vi "CRYDV MARK.vi"(0 "sAction":string="asada", 1 "mVritual_VIRef":refnum<vi>, 2 "sData":string="asada", 3 "MousePos":T1, 4 "DataView Array Index":i32, 5 "SubPanel array":refnum<vi>[](array[refnum]), 6 "Start Pos In":T1) -> (10 "bResult":bool=TRUE)   [LabVIEW 2013]
uses:
  <vilib>/Utility/miscctls.llb/LVRectTypeDef.ctl
  CRYNew View Global.vi
panel:
  in  "Rect_Main":T2
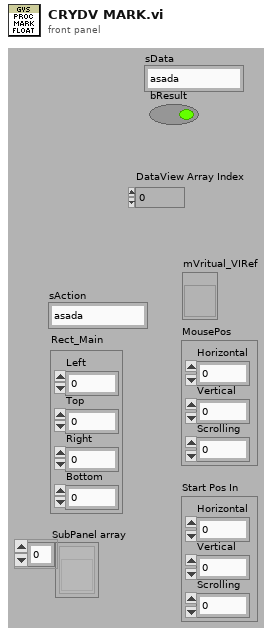
[diagram p1: front panel]
types:
  T1 = cluster{"Horizontal":i32, "Vertical":i32, "Scrolling":i32}
  T2 = typedef "LVRectTypeDef.ctl" = cluster{"Left":i16, "Top":i16, "Right":i16, "Bottom":i16}
  T3 = typedef "Graph Main Info Cluster.ctl" = cluster{"Selected_BarIdx":i32, "Selected_PanelIdx":i32, "Graph Main VIRef":refnum<vi>, "ToolBarClick":bool, "Spliter Ref Array":refnum<vi>[], "Panel Ref Array":refnum<vi>[], "Spliter_matrix":i32[][], "Panel_matrix":i32[][], "child_spliterIdx_matrix":i32[][], "split_pos_matrix":i32[][], "Title State":bool, "sQueueName":string, "Frame nID":i32, "Graph VIRef Array":cluster{"Graph VIRef":refnum<vi>, "Panel Idx":i32, "Frame VIRef":refnum<vi>, "Icon Ring":i32, "Graph Type":string}[], "View Type":string}
  T4 = enum32{"Invalid", "Standard", "Closed", "Hidden", "Minimized", "Maximized"}
  T5 = enum32{"Invalid", "Default", "Floating", "Floating/Auto-Hide", "Modal"}
  T6 = cluster{"Horizontal":bool, "Vertical":bool, "Scrolling":bool}
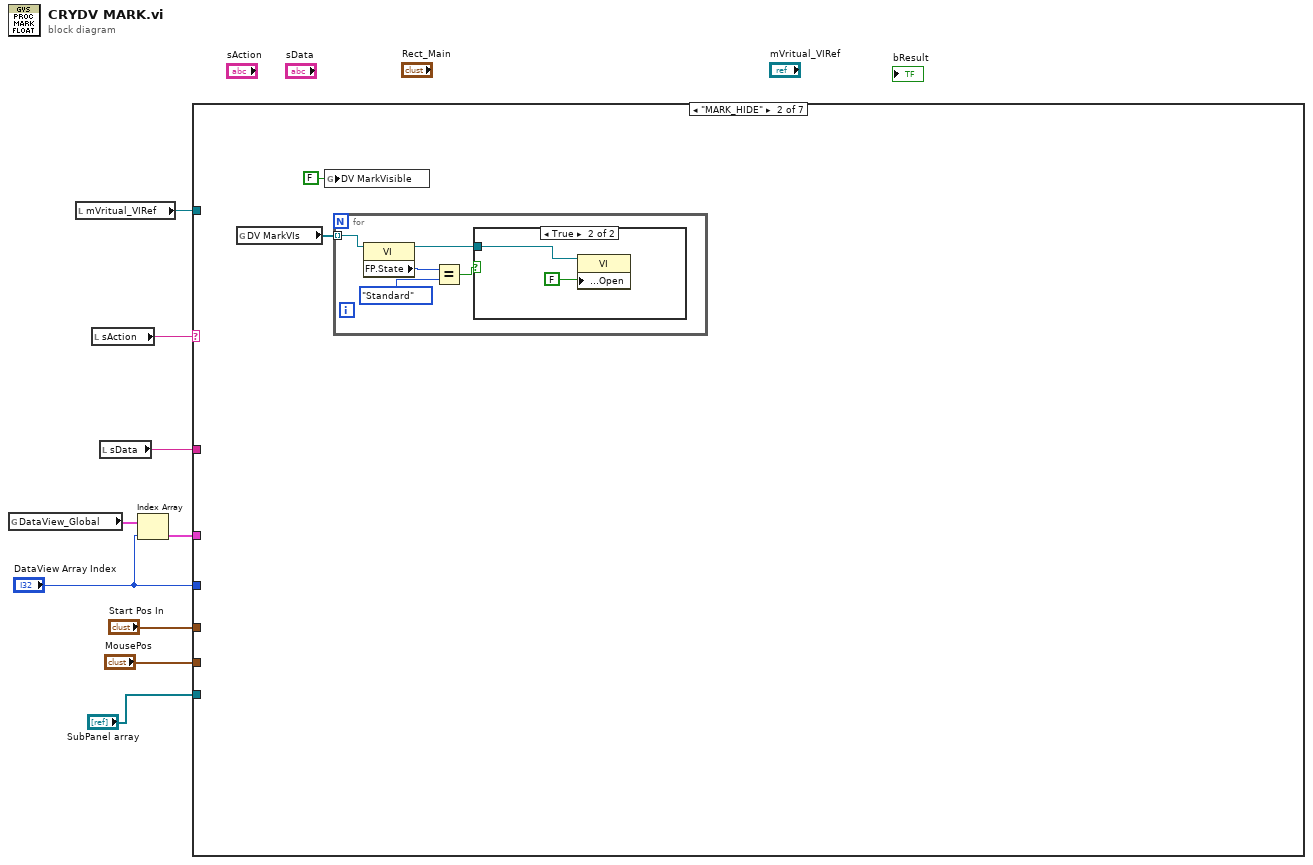
[diagram p0: block diagram]
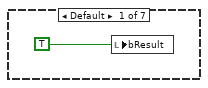
[diagram p2: hidden frame]
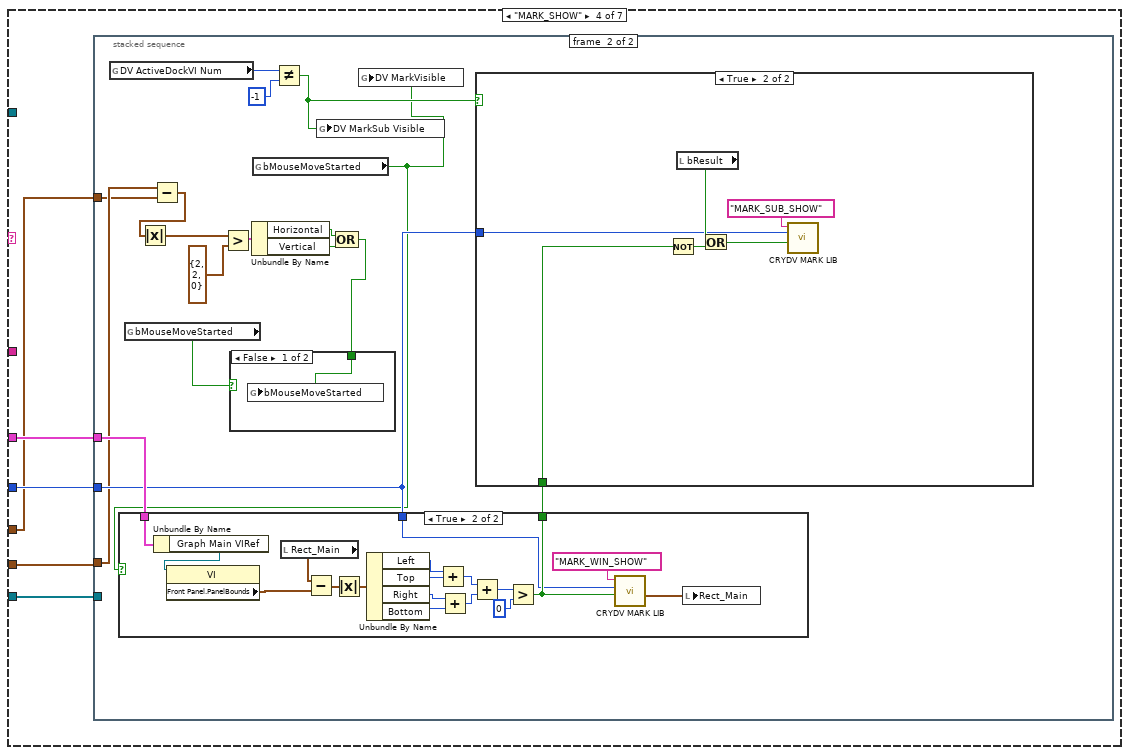
[diagram p5: hidden frame]
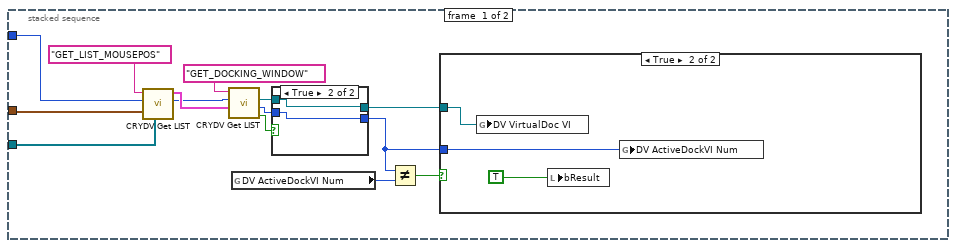
[diagram p6: hidden frame]
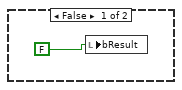
[diagram p7: hidden frame]
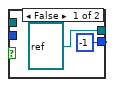
[diagram p8: hidden frame]
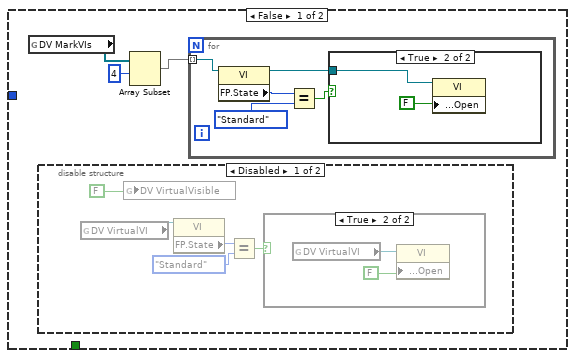
[diagram p11: hidden frame]
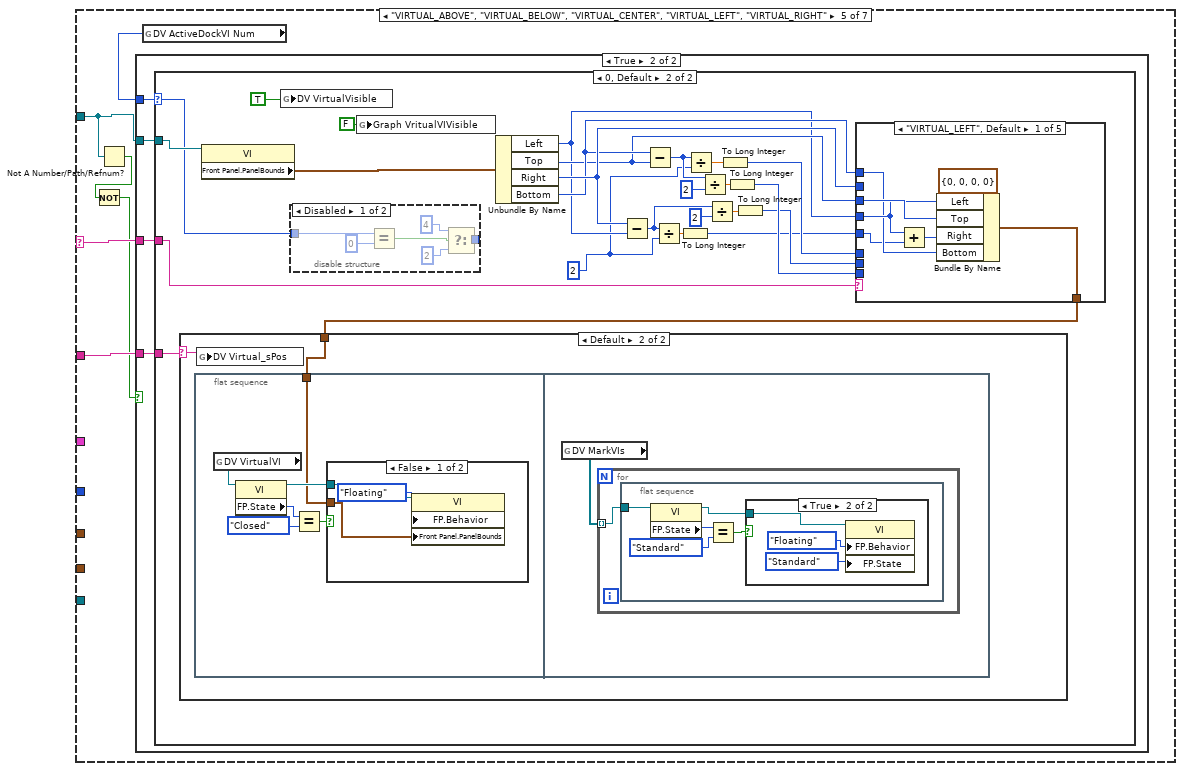
[diagram p15: hidden frame]
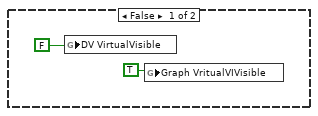
[diagram p16: hidden frame]
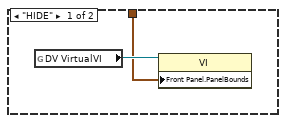
[diagram p19: hidden frame]
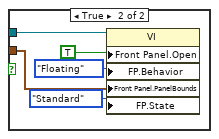
[diagram p20: hidden frame]
diagram:
  n1 = global read "CRYNew View Global.vi" "DataView_Global"() -> (w5:T3[])
  n2 = local read "mVritual_VIRef"() -> (w3:refnum<vi>)
  n3 = local read "sAction"() -> (w9:string)
  n4 = local read "sData"() -> (w8:string)
  n5 = Index Array(array=w5, index="DataView Array Index") -> (element=w7:T3)
  n6 = case shown="\"MARK_HIDE\"" w9 {
    selector: w9 -> [_ _ _ _ w110 _ _]
    tunnel: "MousePos" -> [_ _ _ w24 _ _ w223]
    tunnel: w3 -> [_ _ _ _ w107 _ _]
    tunnel: w8 -> [_ _ _ _ w109 _ _]
    tunnel: w7 -> [_ _ _ w23 _ _ _]
    tunnel: "DataView Array Index" -> [_ _ _ w22 _ _ _]
    tunnel: "SubPanel array" -> [_ _ _ w21 _ _ _]
    tunnel: "Start Pos In" -> [_ _ _ w20 _ _ _]
    frame Default {
      n7 = local write "bResult"(TRUE ("bResult")) -> ()
    }
    frame "MARK_HIDE" {
      n8 = global read "CRYNew View Global.vi" "DV MarkVIs"() -> (w12:refnum<vi>[])
      n9 = global write "CRYNew View Global.vi" "DV MarkVisible"(FALSE ("Mark VI State")) -> ()
      n10 = for {
        tunnel: w12 -> [w15] mode=indexing
        n11 = property class="VI"(reference=w15) -> (reference out=w14:refnum<vi>, "FP.State"=w17:T4)  [unwired: 1 in, 1 out]
        n12 = Equal?(x=w17, y=T4."Standard" ("Front Panel Window:State")) -> (x = y?=w13:bool)
        n13 = case shown="True" w13 {
          tunnel: w14 -> [_ w19]
          frame False {
          }
          frame True {
            n14 = property class="VI"(reference=w19, "Front Panel.Open"=FALSE ("Front Panel Window:Open")) -> ()  [unwired: 1 in, 2 out]
          }
        }
      }
    }
    frame "ADDGRAPHMENU_HIDE" {
    }
    frame "MARK_SHOW" {
      n15 = stacked-sequence {
        tunnel: w24 -> [w37 w50]
        tunnel: w23 -> [_ w59]
        tunnel: w22 -> [w26 w58]
        tunnel: w21 -> [w25 _]
        tunnel: w20 -> [_ w49]
        frame #0 {
          n16 = call "CRYDV Get LIST.vi"("sAction"="GET_LIST_MOUSEPOS", "DataView Array Index"=w26, "MousePos"=w37, "SubPanel array"=w25) -> ("List_Out"=w34:cluster{"nID":i32, "pVIRef":refnum<vi>}[])  [unwired: 1 in, 5 out]
          n17 = call "CRYDV Get LIST.vi"("sAction"="GET_DOCKING_WINDOW", "DataView Array Index"=w26, "List_In"=w34) -> ("pVIRef_Out"=w32:refnum<vi>, "nData_Out"=w29:i32, "bResult"=w33:bool)  [unwired: 2 in, 3 out]
          n18 = global read "CRYNew View Global.vi" "DV ActiveDockVI Num"() -> (w27:i32)
          n19 = case shown="True" w33 {
            tunnel: w32 -> [_ w45]
            tunnel: [-1 w44] -> w30
            tunnel: [refnum<vi> refnum ("Vritual_Docking_VIRef") w45] -> w31
            tunnel: w29 -> [_ w44]
            frame False {
            }
            frame True {
            }
          }
          n20 = Not Equal?(x=w30, y=w27) -> (x != y?=w28:bool)
          n21 = case shown="True" w28 {
            tunnel: w31 -> [_ w41]
            tunnel: w30 -> [_ w39]
            frame False {
              n22 = local write "bResult"(FALSE ("Docking_Update")) -> ()
            }
            frame True {
              n23 = global write "CRYNew View Global.vi" "DV VirtualDoc VI"(w41) -> ()
              n24 = local write "bResult"(TRUE ("Docking_Update")) -> ()
              n25 = global write "CRYNew View Global.vi" "DV ActiveDockVI Num"(w39) -> ()
            }
          }
        }
        frame #1 {
          n26 = global read "CRYNew View Global.vi" "DV ActiveDockVI Num"() -> (w61:i32)
          n27 = global read "CRYNew View Global.vi" "bMouseMoveStarted"() -> (w47:bool)
          n28 = Subtract(x=w50, y=w49) -> (x-y=w52:T1)
          n29 = Absolute Value(x=w52) -> (abs(x)=w51:T1)
          n30 = Greater?(x=w51, y=T1 {"Horizontal"=2, "Vertical"=2, "Scrolling"=0}) -> (0:w55:T6)
          n31 = Unbundle By Name(w55) -> ("Horizontal"=w54:bool, "Vertical"=w53:bool)
          n32 = global read "CRYNew View Global.vi" "bMouseMoveStarted"() -> (w48:bool)
          n33 = case shown="True" w48 {
            tunnel: [_ w66] -> w60
            tunnel: w59 -> [_ w65]
            tunnel: w58 -> [_ w64]
            frame False {
            }
            frame True {
              n34 = Unbundle By Name(w65) -> ("Graph Main VIRef"=w68:refnum<vi>)
              n35 = property class="VI"(reference=w68) -> ("Front Panel.PanelBounds"=w67:T2)  [unwired: 1 in, 2 out]
              n36 = local read "Rect_Main"() -> (w69:T2)
              n37 = Subtract(x=w69, y=w67) -> (x-y=w73:T2)
              n38 = Absolute Value(x=w73) -> (abs(x)=w72:T2)
              n39 = Unbundle By Name(w72) -> ("Left"=w74:i16, "Top"=w77:i16, "Right"=w76:i16, "Bottom"=w75:i16)
              n40 = Add(x=w74, y=w77) -> (x+y=w78:i16)
              n41 = Add(x=w76, y=w75) -> (x+y=w79:i16)
              n42 = Add(x=w78, y=w79) -> (x+y=w71:i16)
              n43 = Greater?(x=w71, y=0) -> (0:w66:bool)
              n44 = call "CRYDV MARK LIB.vi"("sAction"="MARK_WIN_SHOW", "DataView Array Index"=w64, "Docking_Update"=w66) -> ("Rect_Out"=w80:T2)  [unwired: 1 in, 6 out]
              n45 = local write "Rect_Main"(w80) -> ()
            }
          }
          n46 = Not Equal?(x=w61, y=-1) -> (x != y?=w57:bool)
          n47 = global write "CRYNew View Global.vi" "DV MarkSub Visible"(w57) -> ()
          n48 = Compound Arithmetic op=OR(w54, w53) -> (w46:bool)
          n49 = case shown="False" w47 {
            tunnel: w46 -> [w63 _]
            frame False {
              n50 = global write "CRYNew View Global.vi" "bMouseMoveStarted"(w63) -> ()
            }
            frame True {
            }
          }
          n51 = global write "CRYNew View Global.vi" "DV MarkVisible"(w48) -> ()
          n52 = case shown="True" w57 {
            tunnel: w60 -> [_ w100]
            tunnel: w58 -> [_ w99]
            frame False {
              n53 = global read "CRYNew View Global.vi" "DV MarkVIs"() -> (w84:refnum<vi>[])
              n54 = disable-structure shown="Disabled" {
                frame Disabled {
                  n55 = global read "CRYNew View Global.vi" "DV VirtualVI"() -> (w87:refnum<vi>)
                  n56 = global write "CRYNew View Global.vi" "DV VirtualVisible"(FALSE ("VirtualVi")) -> ()
                  n57 = property class="VI"(reference=w87) -> ("FP.State"=w88:T4)  [unwired: 1 in, 2 out]
                  n58 = Equal?(x=w88, y=T4."Standard" ("Front Panel Window:State")) -> (x = y?=w85:bool)
                  n59 = case shown="True" w85 {
                    frame False {
                    }
                    frame True {
                      n60 = global read "CRYNew View Global.vi" "DV VirtualVI"() -> (w90:refnum<vi>)
                      n61 = property class="VI"(reference=w90, "Front Panel.Open"=FALSE ("Front Panel Window:Open")) -> ()  [unwired: 1 in, 2 out]
                    }
                  }
                }
                frame Enabled {
                }
              }
              n62 = Array Subset(array=w84, index=4) -> (w83:refnum<vi>[])  [unwired: 1 in]
              n63 = for {
                tunnel: w83 -> [w94] mode=indexing
                n64 = property class="VI"(reference=w94) -> (reference out=w93:refnum<vi>, "FP.State"=w96:T4)  [unwired: 1 in, 1 out]
                n65 = Equal?(x=w96, y=T4."Standard" ("Front Panel Window:State")) -> (x = y?=w92:bool)
                n66 = case shown="True" w92 {
                  tunnel: w93 -> [_ w98]
                  frame False {
                  }
                  frame True {
                    n67 = property class="VI"(reference=w98, "Front Panel.Open"=FALSE ("Front Panel Window:Open")) -> ()  [unwired: 1 in, 2 out]
                  }
                }
              }
            }
            frame True {
              n68 = Not(x=w100) -> (.not. x?=w102:bool)
              n69 = local read "bResult"() -> (w103:bool)
              n70 = Or(x=w103, y=w102) -> (x .or. y?=w104:bool)
              n71 = call "CRYDV MARK LIB.vi"("sAction"="MARK_SUB_SHOW", "DataView Array Index"=w99, "Docking_Update"=w104) -> ()  [unwired: 1 in, 7 out]
            }
          }
        }
      }
    }
    frame "VIRTUAL_ABOVE", "VIRTUAL_BELOW", "VIRTUAL_CENTER", "VIRTUAL_LEFT", "VIRTUAL_RIGHT" {
      n72 = Not A Number/Path/Refnum?(number/path/refnum=w107) -> (NaN/Path/Refnum?=w106:bool)
      n73 = Not(x=w106) -> (.not. x?=w105:bool)
      n74 = global read "CRYNew View Global.vi" "DV ActiveDockVI Num"() -> (w108:i32)
      n75 = case shown="True" w105 {
        tunnel: w107 -> [_ w116]
        tunnel: w110 -> [_ w115]
        tunnel: w109 -> [_ w114]
        tunnel: w108 -> [_ w113]
        frame False {
          n76 = global write "CRYNew View Global.vi" "DV VirtualVisible"(FALSE ("Virtual_State_Up")) -> ()
          n77 = global write "CRYNew View Global.vi" "Graph VritualVIVisible"(TRUE ("VritualVIVisible")) -> ()
        }
        frame True {
          n78 = case shown="0, Default" w113 {
            selector: w113 -> [_ w120]
            tunnel: w115 -> [_ w130]
            tunnel: w116 -> [_ w140]
            tunnel: w114 -> [_ w121]
            frame -1 {
            }
            frame 0, Default {
              w118 = 2
              n79 = property class="VI"(reference=w140) -> ("Front Panel.PanelBounds"=w119:T2)  [unwired: 1 in, 2 out]
              n80 = global write "CRYNew View Global.vi" "DV VirtualVisible"(TRUE ("Virtual_State_Up")) -> ()
              n81 = disable-structure shown="Disabled" {
                disable-tunnel: [w145 _] -> _
                disable-tunnel: w120 -> [w142 _]
                frame Disabled {
                  n82 = Equal?(x=w142, y=0) -> (x = y?=w143:bool)
                  n83 = Select(t=4, s=w143, f=2) -> (s? t:f=w145:i32)
                }
                frame Enabled {
                }
              }
              n84 = global write "CRYNew View Global.vi" "Graph VritualVIVisible"(FALSE ("VritualVIVisible")) -> ()
              n85 = Unbundle By Name(w119) -> ("Left"=w132:i16, "Top"=w133:i16, "Right"=w139:i16, "Bottom"=w138:i16)
              n86 = Subtract(x=w139, y=w132) -> (x-y=w134:i16)
              n87 = Subtract(x=w138, y=w133) -> (x-y=w137:i16)
              n88 = Divide(x=w134, y=w118) -> (x/y=w123:dbl)
              n89 = To Long Integer(number=w123) -> (32bit integer=w122:i32)
              n90 = Divide(x=w137, y=w118) -> (x/y=w129:dbl)
              n91 = Divide(x=w137, y=2) -> (x/y=w127:dbl)
              n92 = Divide(x=w134, y=2) -> (x/y=w125:dbl)
              n93 = To Long Integer(number=w129) -> (32bit integer=w128:i32)
              n94 = To Long Integer(number=w127) -> (32bit integer=w126:i32)
              n95 = To Long Integer(number=w125) -> (32bit integer=w124:i32)
              n96 = case shown="\"VIRTUAL_LEFT\", Default" w130 {
                tunnel: w132 -> [w180 _ w194 w201 w216]
                tunnel: w133 -> [w181 w188 w193 _ w215]
                tunnel: w139 -> [_ w186 w195 w202 _]
                tunnel: w138 -> [w178 w187 _ w199 _]
                tunnel: w122 -> [w177 w185 _ _ w207]
                tunnel: [w176 w183 w190 w197 w204] -> w141
                tunnel: w128 -> [_ _ w192 w200 w208]
                tunnel: w124 -> [_ _ _ _ w210]
                tunnel: w126 -> [_ _ _ _ w209]
                frame "VIRTUAL_LEFT", Default {
                  n97 = Add(x=w180, y=w177) -> (x+y=w179:i32)
                  n98 = Bundle By Name(cluster=T2 {"Left"=0, "Top"=0, "Right"=0, "Bottom"=0} ("Front Panel Window:Panel Bounds"), "Left"=w180, "Top"=w181, "Right"=w179, "Bottom"=w178) -> (w176:T2)
                }
                frame "VIRTUAL_RIGHT" {
                  n99 = Subtract(x=w186, y=w185) -> (x-y=w184:i32)
                  n100 = Bundle By Name(cluster=T2 {"Left"=0, "Top"=0, "Right"=0, "Bottom"=0} ("Front Panel Window:Panel Bounds"), "Left"=w184, "Top"=w188, "Right"=w186, "Bottom"=w187) -> (w183:T2)
                }
                frame "VIRTUAL_ABOVE" {
                  n101 = Add(x=w193, y=w192) -> (x+y=w191:i32)
                  n102 = Bundle By Name(cluster=T2 {"Left"=0, "Top"=0, "Right"=0, "Bottom"=0} ("Front Panel Window:Panel Bounds"), "Left"=w194, "Top"=w193, "Right"=w195, "Bottom"=w191) -> (w190:T2)
                }
                frame "VIRTUAL_BELOW" {
                  n103 = Subtract(x=w199, y=w200) -> (x-y=w198:i32)
                  n104 = Bundle By Name(cluster=T2 {"Left"=0, "Top"=0, "Right"=0, "Bottom"=0} ("Front Panel Window:Panel Bounds"), "Left"=w201, "Top"=w198, "Right"=w202, "Bottom"=w199) -> (w197:T2)
                }
                frame "VIRTUAL_CENTER" {
                  n105 = Add(x=w210, y=w216) -> (x+y=w206:i32)
                  n106 = Add(x=w209, y=w215) -> (x+y=w205:i32)
                  n107 = Subtract(x=w206, y=w207) -> (x-y=w214:i32)
                  n108 = Subtract(x=w205, y=w208) -> (x-y=w213:i32)
                  n109 = Add(x=w206, y=w207) -> (x+y=w212:i32)
                  n110 = Add(x=w205, y=w208) -> (x+y=w211:i32)
                  n111 = Bundle By Name(cluster=T2 {"Left"=0, "Top"=0, "Right"=0, "Bottom"=0} ("Front Panel Window:Panel Bounds"), "Left"=w214, "Top"=w213, "Right"=w212, "Bottom"=w211) -> (w204:T2)
                }
              }
              n112 = case shown="Default" w121 {
                selector: w121 -> [_ w150]
                tunnel: w141 -> [w148 w151]
                frame "HIDE" {
                  n113 = global read "CRYNew View Global.vi" "DV VirtualVI"() -> (w149:refnum<vi>)
                  n114 = property class="VI"(reference=w149, "Front Panel.PanelBounds"=w148) -> ()  [unwired: 1 in, 2 out]
                }
                frame Default {
                  n115 = flat-sequence {
                    tunnel: w151 -> [w154]
                    frame #0 {
                      n116 = global read "CRYNew View Global.vi" "DV VirtualVI"() -> (w153:refnum<vi>)
                      n117 = property class="VI"(reference=w153) -> (reference out=w157:refnum<vi>, "FP.State"=w155:T4)  [unwired: 1 in, 1 out]
                      n118 = Equal?(x=w155, y=T4."Closed" ("Front Panel Window:State")) -> (x = y?=w152:bool)
                      n119 = case shown="False" w152 {
                        tunnel: w154 -> [w158 w165]
                        tunnel: w157 -> [w160 w162]
                        frame False {
                          n120 = property class="VI"(reference=w160, "FP.Behavior"=T5."Floating" ("Front Panel Window:Behavior"), "Front Panel.PanelBounds"=w158) -> ()  [unwired: 1 in, 2 out]
                        }
                        frame True {
                          n121 = property class="VI"(reference=w162, "Front Panel.Open"=TRUE ("Front Panel Window:Open"), "FP.Behavior"=T5."Floating" ("Front Panel Window:Behavior"), "Front Panel.PanelBounds"=w165, "FP.State"=T4."Standard" ("Front Panel Window:State")) -> ()  [unwired: 1 in, 2 out]
                        }
                      }
                    }
                    frame #1 {
                      n122 = global read "CRYNew View Global.vi" "DV MarkVIs"() -> (w166:refnum<vi>[])
                      n123 = for {
                        tunnel: w166 -> [w167] mode=indexing
                        n124 = flat-sequence {
                          tunnel: w167 -> [w172]
                          frame #0 {
                            n125 = property class="VI"(reference=w172) -> (reference out=w169:refnum<vi>, "FP.State"=w171:T4)  [unwired: 1 in, 1 out]
                            n126 = Equal?(x=w171, y=T4."Standard" ("Front Panel Window:State")) -> (x = y?=w168:bool)
                            n127 = case shown="True" w168 {
                              tunnel: w169 -> [_ w173]
                              frame False {
                              }
                              frame True {
                                n128 = property class="VI"(reference=w173, "FP.Behavior"=T5."Floating" ("Front Panel Window:Behavior"), "FP.State"=T4."Standard" ("Front Panel Window:State")) -> ()  [unwired: 1 in, 2 out]
                              }
                            }
                          }
                        }
                      }
                    }
                  }
                  n129 = global write "CRYNew View Global.vi" "DV Virtual_sPos"(w150) -> ()
                }
              }
            }
          }
        }
      }
    }
    frame "VIRTUAL_HIDE" {
      n130 = global write "CRYNew View Global.vi" "DV VirtualVisible"(FALSE ("VirtualVi")) -> ()
      n131 = global write "CRYNew View Global.vi" "DV Virtual_sPos"("" ("Virtual_sPos")) -> ()
      n132 = global read "CRYNew View Global.vi" "DV VirtualVI"() -> (w219:refnum<vi>)
      n133 = property class="VI"(reference=w219, "Front Panel.Open"=FALSE ("Front Panel Window:Open")) -> ()  [unwired: 1 in, 2 out]
    }
    frame "CHECK_INMARK" {
      n134 = global read "CRYNew View Global.vi" "DV MarkVIs"() -> (w222:refnum<vi>[])
      n135 = for {
        tunnel: w222 -> [w241] mode=indexing
        tunnel: w223 -> [w239]
        tunnel: [w225] -> w224
        stop <- w225 stop-if-true
        n136 = Unbundle By Name(w239) -> ("Horizontal"=w238:i32, "Vertical"=w229:i32)
        n137 = property class="VI"(reference=w241) -> ("Front Panel.PanelBounds"=w240:T2)  [unwired: 1 in, 2 out]
        n138 = Unbundle By Name(w240) -> ("Left"=w237:i16, "Right"=w236:i16, "Top"=w235:i16, "Bottom"=w234:i16)
        n139 = Less?(x=w238, y=w237) -> (x < y?=w233:bool)
        n140 = Greater?(x=w238, y=w236) -> (0:w231:bool)
        n141 = Less?(x=w229, y=w235) -> (x < y?=w232:bool)
        n142 = Greater?(x=w229, y=w234) -> (0:w230:bool)
        n143 = Or(x=w233, y=w231) -> (x .or. y?=w227:bool)
        n144 = Or(x=w232, y=w230) -> (x .or. y?=w228:bool)
        n145 = Or(x=w227, y=w228) -> (x .or. y?=w226:bool)
        n146 = Not(x=w226) -> (.not. x?=w225:bool)
      }
      n147 = local write "bResult"(w224) -> ()
    }
  }
